vi "Stop Core.vi"(10 "final error code":i32, 11 "Actor Monitor in":refnum<class "Actor Monitor.lvclass">) -> (3 "Actor Monitor out":refnum<class "Actor Monitor.lvclass">)   [LabVIEW 2018, in "Monitored Actor.lvlib" / "Actor Monitor.lvclass"]
doc: "Stops the periodic poller\n\nCopyright: MGI\nAuthored by: Derek Trepanier"
uses:
  Actor Monitor.lvclass
  Actor Monitor.lvclass/Actor Monitor.ctl
  <vilib>/ActorFramework/Actor/Actor.lvclass
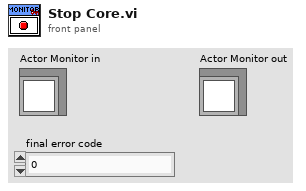
[diagram p1: front panel]
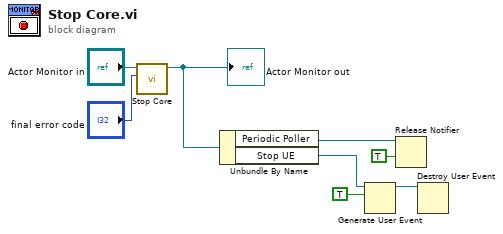
[diagram p0: block diagram]
diagram:
  n1 = call-parent "Stop Core.vi"("final error code"="final error code", "Actor in"="Actor Monitor in") -> ("Actor out"=w6:refnum<class "Actor Monitor.lvclass">)  [unwired: 9 in]
  "Actor Monitor out" <- w6
  n2 = Unbundle By Name(w6) -> ("Periodic Poller"=w5:refnum<notifier>, "Stop UE"=w2:refnum<user-event>)
  n3 = Generate User Event(user event=w2, event data cluster=TRUE ("event data")) -> (user event out=w3:refnum<user-event>)  [unwired: 2 in, 1 out]
  n4 = Release Notifier(notifier=w5, force destroy? (F)=TRUE) -> ()  [unwired: 1 in, 3 out]
  n5 = Destroy User Event(user event=w3) -> ()  [unwired: 1 in, 1 out]
